vi "BASE-Main.vi"() -> ()   [LabVIEW 2017]
uses:
  <vilib>/Utility/error.llb/DialogType.ctl
  55ed0eea-cd20-493f-8468-85b8c1a0a0c0.vi
panel:
  out "Status Number":i32
  out "Status":i32(ring)=1 items=["Stopped"=1, "StartPending"=2, "StopPending"=3, "Running"=4, "ContinuePending"=5, "PausePending"=6, "Paused"=7]
  in  "RECIPE":bool
  out "error out":errorcluster
  in  "Logout":bool
  in  "Stop":bool
  in  "Create Login":bool
  in  "Reports":bool
  in  "Start":bool
  out "Time":string
  out "Date":string
  in  "Login":bool
  # "Machine Name"
  # "UNIQUE CIRCLE\nAUTOMATION Pvt Ltd"
types:
  T1 = enum8{"Enabled", "Disabled", "Disabled and Grayed Out"}
  T2 = typedef "DialogType.ctl" = u16
  T3 = enum32{"Invalid", "Standard", "Closed", "Hidden", "Minimized", "Maximized"}
  T4 = enum32{"invalid app kind", "Development System", "Run Time System", "Student Edition", "Embedded LabVIEW", "Evaluation", "Custom"}
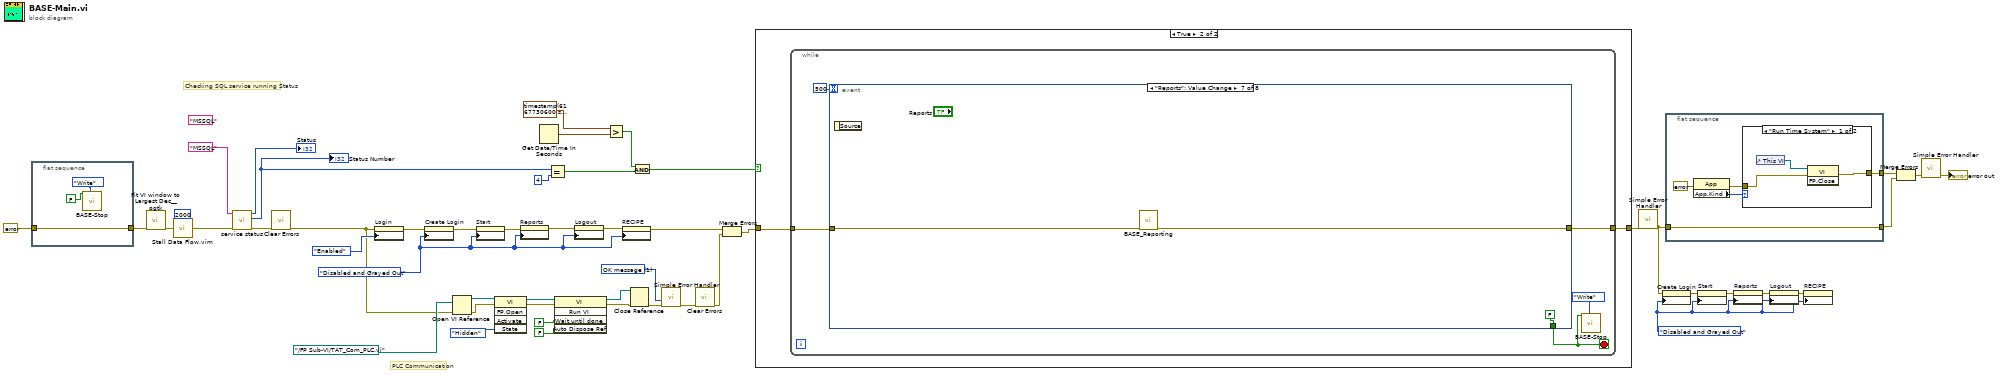
[diagram p0: block diagram]
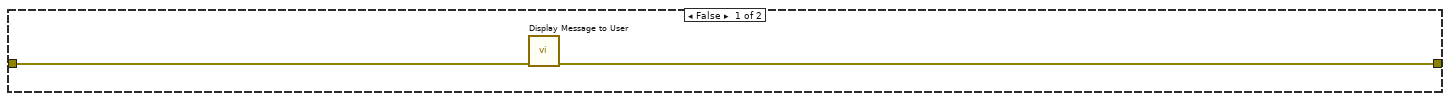
[diagram p3: hidden frame]
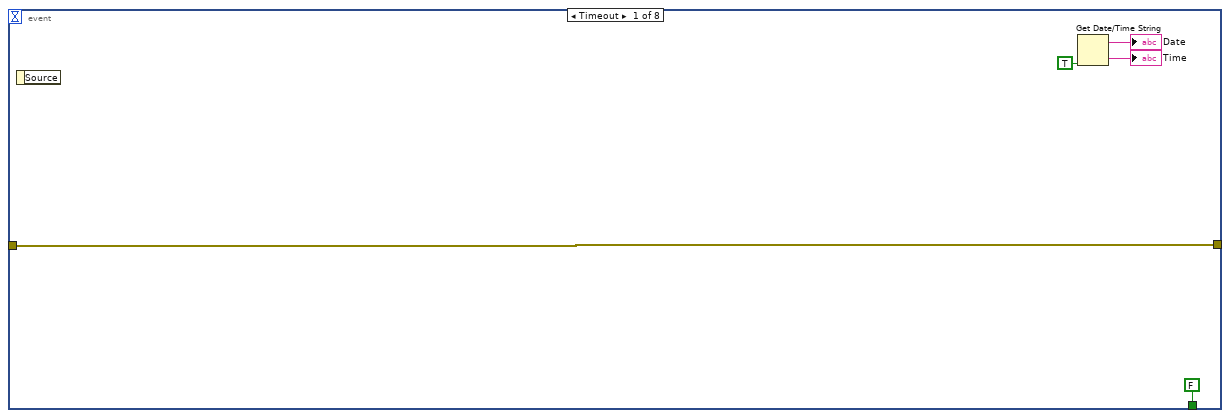
[diagram p4: hidden frame]
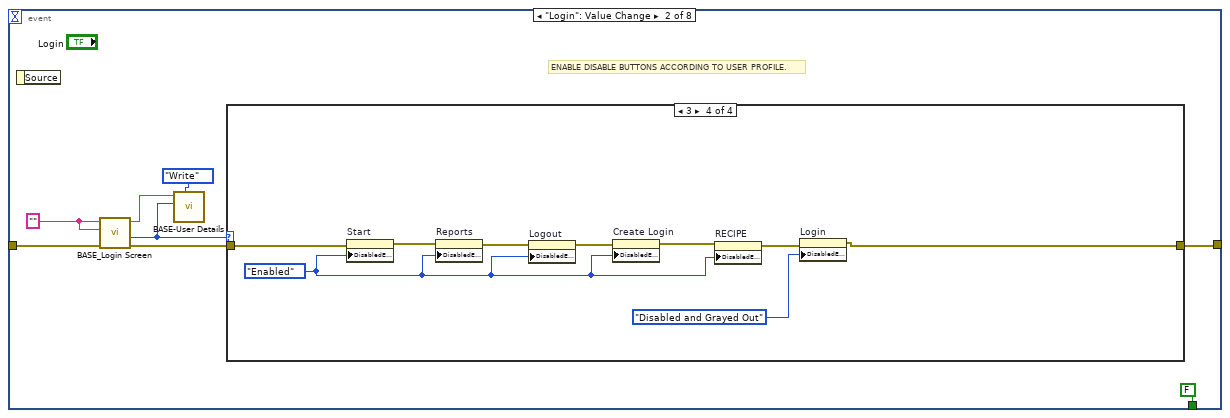
[diagram p5: hidden frame]
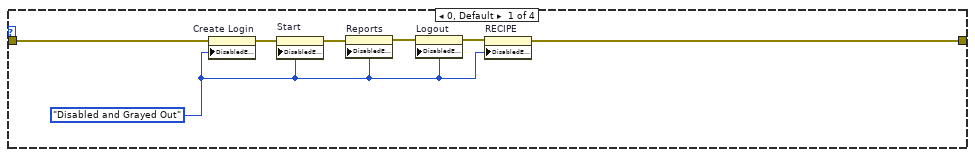
[diagram p6: hidden frame]
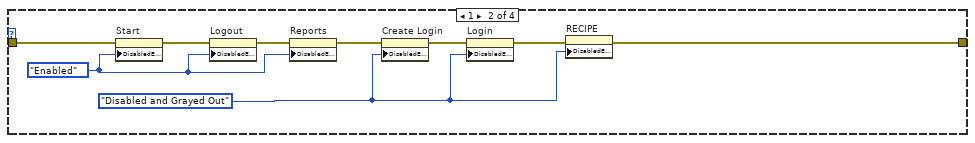
[diagram p7: hidden frame]
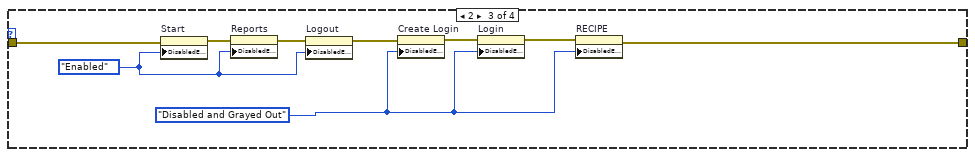
[diagram p8: hidden frame]
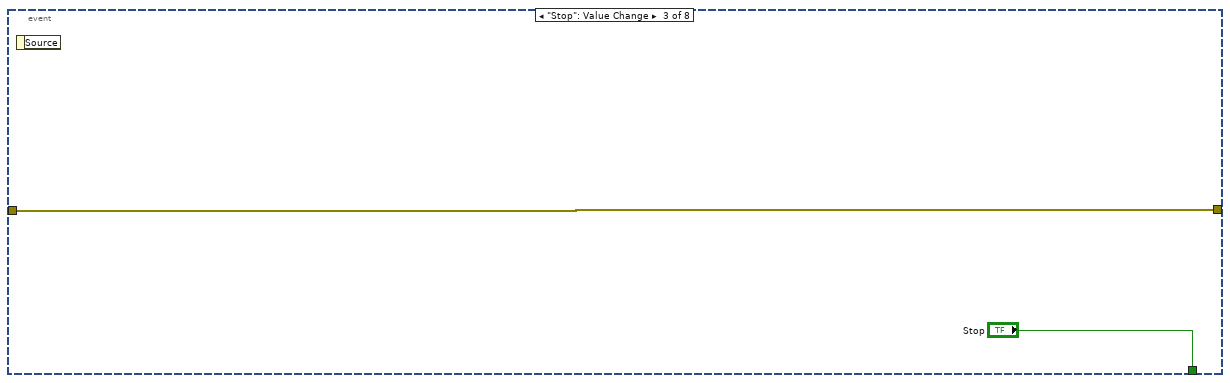
[diagram p9: hidden frame]
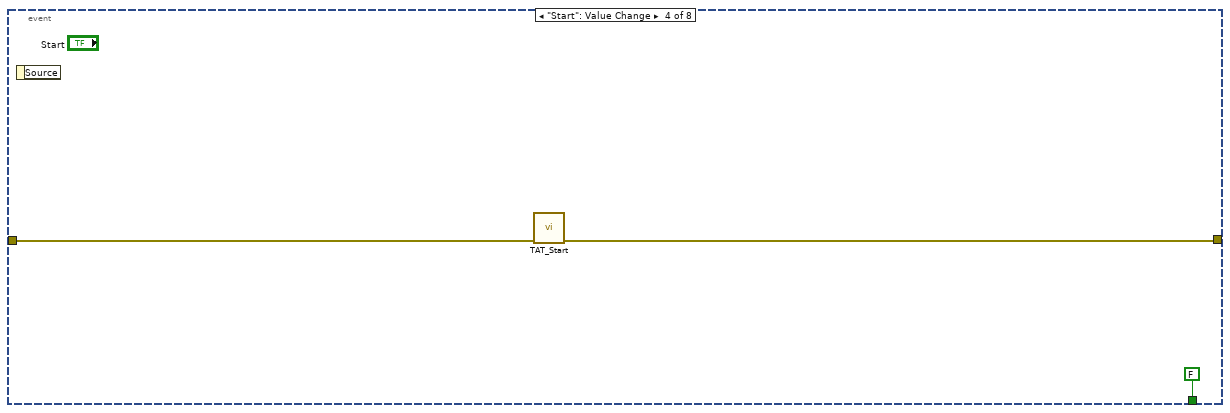
[diagram p10: hidden frame]
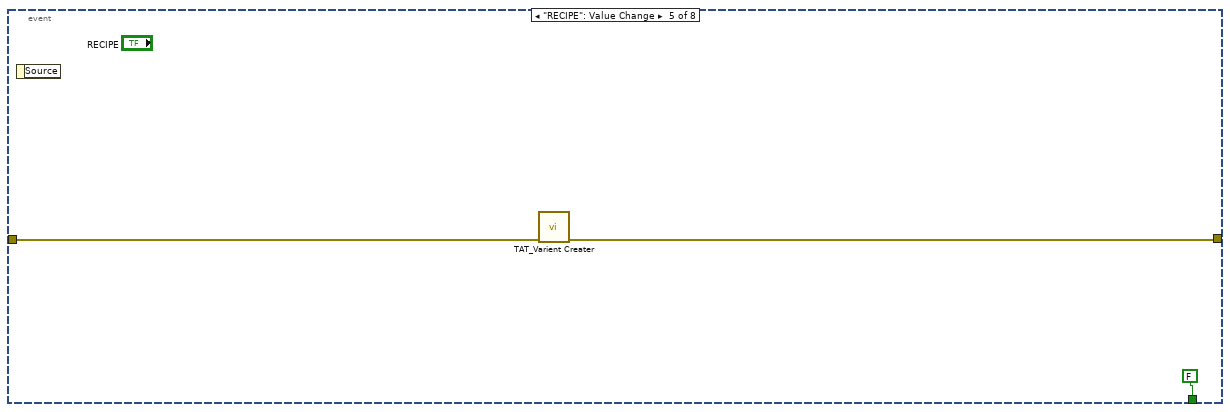
[diagram p11: hidden frame]
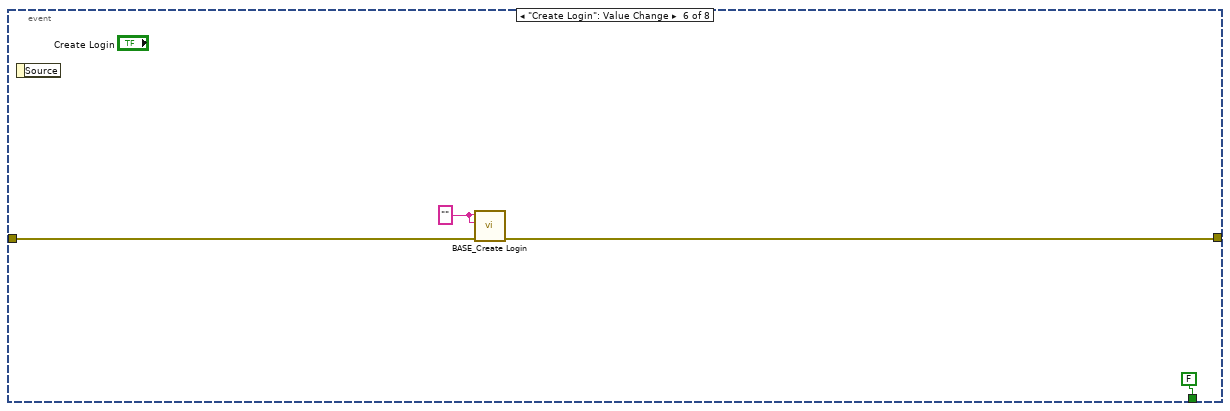
[diagram p12: hidden frame]
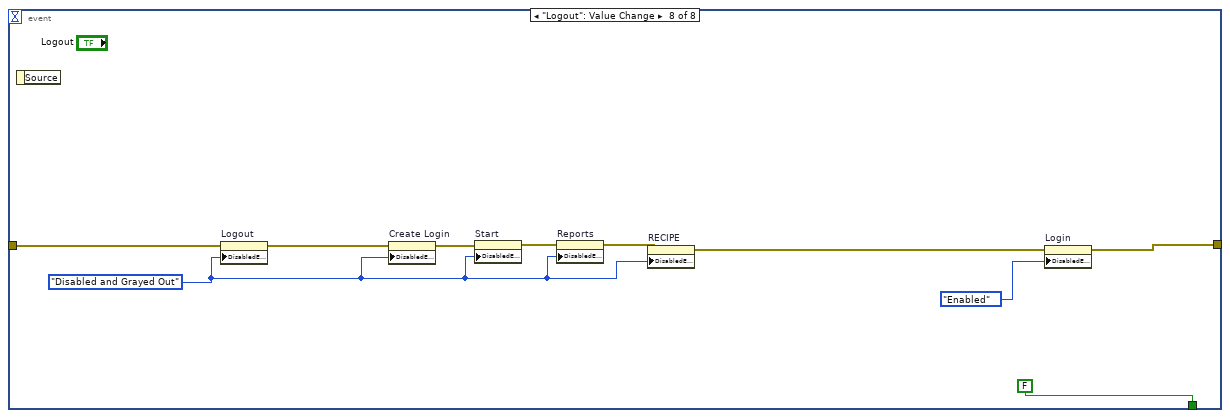
[diagram p13: hidden frame]
diagram:
  w7 = T1."Disabled and Grayed Out" ("Disabled")
  (unwired) "MSSQL" ("Service Name")
  w28 = T2 1 items=["no dialog", "OK message", "continue or stop message", "OK message + warnings", "continue/stop + warnings"] ("type of dialog (OK msg:1)")
  w8 = T1."Disabled and Grayed Out" ("Disabled")
  # "PLC Communication"
  # "Checking SQL service running Status"
  n1 = flat-sequence {
    tunnel: [w53] -> w41
    tunnel: errorcluster {"status"=FALSE, "code"=0, "source"=""} ("error constant") -> [w53]
    frame #0 {
      n2 = call "BASE-Stop.vi"("Enum"=enum16{"Read", "Write"}."Write", "Stop"=FALSE) -> ()  [unwired: 9 in, 1 out]
    }
  }
  n3 = call <userlib>:"Fit VI window to Largest Dec__ogtk.vi"("error in (no error)"=w41) -> ("error out"=w13:errorcluster)  [unwired: 5 in, 1 out]
  n4 = call "Stall Data Flow.vim"("value in"=w13, "milliseconds to wait"=u32 2000) -> ("value out"=w12:errorcluster)  [unwired: 1 out]
  n5 = call "service status.vi"("error in"=w12, "Service Name"="MSSQL") -> ("error out"=w20:errorcluster, "Status Number"=w22:i32, "Status"=→"Status":i32)  [unwired: 6 in, 1 out]
  "Status Number" <- w22
  n6 = call <vilib>:"Clear Errors.vi"("error in (no error)"=w20) -> ("error out"=w19:errorcluster)  [unwired: 5 in, 1 out]
  n7 = property on="Login" class="Bool"(error in=w19, "DisabledEnum"=T1."Enabled" ("Disabled")) -> (error out=w45:errorcluster)  [unwired: 1 in, 1 out]
  n8 = property on="Create Login" class="Bool"(error in=w45, "DisabledEnum"=w8) -> (error out=w49:errorcluster)  [unwired: 1 in, 1 out]
  n9 = Open VI Reference(vi path=path "../FP Sub-VI/TAT_Com_PLC.vi", error in (no error)=w19) -> (vi reference=w37:refnum<vi>, error out=w38:errorcluster)  [unwired: 4 in]
  n10 = property on="Start" class="Bool"(error in=w49, "DisabledEnum"=w8) -> (error out=w9:errorcluster)  [unwired: 1 in, 1 out]
  n11 = invoke class="VI" method="FP.Open"(reference=w37, error in=w38, "State"=T3."Hidden") -> (reference out=w40:refnum<vi>, error out=w39:errorcluster)  [unwired: 2 in, 3 out]
  n12 = property on="Reports" class="Bool"(error in=w9, "DisabledEnum"=w8) -> (error out=w43:errorcluster)  [unwired: 1 in, 1 out]
  n13 = Get Date/Time In Seconds() -> (seconds since 1Jan1904=w15:timestamp)
  n14 = Equal?(x=w22, y=4) -> (x = y?=w18:bool)
  n15 = invoke class="VI" method="Run VI"(reference=w40, error in=w39, "Wait until done"=FALSE ("Wait Until Done"), "Auto Dispose Ref"=FALSE ("Auto Dispose Reference")) -> (reference out=w36:refnum<vi>, error out=w35:errorcluster)  [unwired: 1 in, 3 out]
  n16 = property on="Logout" class="Bool"(error in=w43, "DisabledEnum"=w8) -> (error out=w10:errorcluster)  [unwired: 1 in, 1 out]
  n17 = Greater?(x=timestamp(6167730600 s since 1904-01-01), y=w15) -> (0:w14:bool)
  n18 = property on="RECIPE" class="Bool"(error in=w10, "DisabledEnum"=w8) -> (error out=w1:errorcluster)  [unwired: 1 in, 1 out]
  n19 = Close Reference(reference=w36, error in (no error)=w35) -> (error out=w29:errorcluster)
  n20 = And(x=w14, y=w18) -> (x .and. y?=w17:bool)
  n21 = call <vilib>:"Simple Error Handler.vi"("type of dialog (OK msg:1)"=w28, "error in (no error)"=w29) -> ("error out"=w27:errorcluster)  [unwired: 3 in, 4 out]
  n22 = call <vilib>:"Clear Errors.vi"("error in (no error)"=w27) -> ("error out"=w26:errorcluster)  [unwired: 5 in, 1 out]
  n23 = Merge Errors(w1, w26) -> (w31:errorcluster)
  n24 = case shown="True" w17 {
    tunnel: w31 -> [w55 w57]
    tunnel: [w54 w56] -> w50
    frame False {
      n25 = call "Display Message to User"("error in (no error)"=w55) -> ("error out"=w54:errorcluster)  [unwired: 9 in, 1 out]
    }
    frame True {
      n26 = while {
        tunnel: w57 -> [w61]
        tunnel: [w60] -> w56
        stop <- w58 stop-if-true
        n27 = event shown="[6] \"Reports\": Value Change" {
          selector: _ -> [_ _ _ _ _ _ _ _]
          dyn-events: _ -> [_ _ _ _ _ _ _ _]
          timeout: 500 -> [_ _ _ _ _ _ _ _]
          tunnel: w61 -> [w65 w75 w110 w113 w116 w121 w123 w131]
          tunnel: [w65 w68 w110 w112 w115 w120 w122 w132] -> w60
          tunnel: [FALSE ("Stop") FALSE ("Stop") "Stop" FALSE ("Stop") FALSE ("Stop") FALSE ("Stop") FALSE ("Stop") FALSE ("Stop")] -> w58
          event Timeout {
            n28 = event-data() -> ()  [unwired: 1 in, 1 out]
            n29 = Get Date/Time String(want seconds? (F)=TRUE) -> (date string=→"Date":string, time string=→"Time":string)  [unwired: 2 in]
          }
          event "Login": Value Change {
            w71 = "" ("User Name")
            # "ENABLE DISABLE BUTTONS ACCORDING TO USER PROFILE."
            n30 = event-data() -> ()  [unwired: 1 in, 1 out]
            n31 = call "BASE_Login Screen.vi"("Error In"=w75, "Password"=w71, "User Name"=w71) -> ("error out"=w74:errorcluster, "Level"=w69:i32, "User Name Out"=w72:string)  [unwired: 5 in, 1 out]
            n32 = call "BASE-User Details.vi"("Enum"=enum16{"Read", "Write"}."Write", "Level In"=w69, "User Name In"=w72) -> ()  [unwired: 7 in, 2 out]
            n33 = case shown="3" w69 {
              tunnel: w74 -> [w80 w91 w100 w109]
              tunnel: [w76 w83 w92 w101] -> w68
              frame 0, Default {
                w77 = T1."Disabled and Grayed Out" ("Disabled")
                n34 = property on="Create Login" class="Bool"(error in=w80, "DisabledEnum"=w77) -> (error out=w82:errorcluster)  [unwired: 1 in, 1 out]
                n35 = property on="Start" class="Bool"(error in=w82, "DisabledEnum"=w77) -> (error out=w81:errorcluster)  [unwired: 1 in, 1 out]
                n36 = property on="Reports" class="Bool"(error in=w81, "DisabledEnum"=w77) -> (error out=w78:errorcluster)  [unwired: 1 in, 1 out]
                n37 = property on="Logout" class="Bool"(error in=w78, "DisabledEnum"=w77) -> (error out=w79:errorcluster)  [unwired: 1 in, 1 out]
                n38 = property on="RECIPE" class="Bool"(error in=w79, "DisabledEnum"=w77) -> (error out=w76:errorcluster)  [unwired: 1 in, 1 out]
              }
              frame 1 {
                w85 = T1."Disabled and Grayed Out" ("Disabled")
                w84 = T1."Enabled" ("Disabled")
                n39 = property on="Start" class="Bool"(error in=w91, "DisabledEnum"=w84) -> (error out=w87:errorcluster)  [unwired: 1 in, 1 out]
                n40 = property on="Logout" class="Bool"(error in=w87, "DisabledEnum"=w84) -> (error out=w89:errorcluster)  [unwired: 1 in, 1 out]
                n41 = property on="Reports" class="Bool"(error in=w89, "DisabledEnum"=w84) -> (error out=w90:errorcluster)  [unwired: 1 in, 1 out]
                n42 = property on="Create Login" class="Bool"(error in=w90, "DisabledEnum"=w85) -> (error out=w88:errorcluster)  [unwired: 1 in, 1 out]
                n43 = property on="Login" class="Bool"(error in=w88, "DisabledEnum"=w85) -> (error out=w86:errorcluster)  [unwired: 1 in, 1 out]
                n44 = property on="RECIPE" class="Bool"(error in=w86, "DisabledEnum"=w85) -> (error out=w83:errorcluster)  [unwired: 1 in, 1 out]
              }
              frame 2 {
                w93 = T1."Disabled and Grayed Out" ("Disabled")
                w94 = T1."Enabled" ("Disabled")
                n45 = property on="Start" class="Bool"(error in=w100, "DisabledEnum"=w94) -> (error out=w97:errorcluster)  [unwired: 1 in, 1 out]
                n46 = property on="Reports" class="Bool"(error in=w97, "DisabledEnum"=w94) -> (error out=w99:errorcluster)  [unwired: 1 in, 1 out]
                n47 = property on="Logout" class="Bool"(error in=w99, "DisabledEnum"=w94) -> (error out=w95:errorcluster)  [unwired: 1 in, 1 out]
                n48 = property on="Create Login" class="Bool"(error in=w95, "DisabledEnum"=w93) -> (error out=w98:errorcluster)  [unwired: 1 in, 1 out]
                n49 = property on="Login" class="Bool"(error in=w98, "DisabledEnum"=w93) -> (error out=w96:errorcluster)  [unwired: 1 in, 1 out]
                n50 = property on="RECIPE" class="Bool"(error in=w96, "DisabledEnum"=w93) -> (error out=w92:errorcluster)  [unwired: 1 in, 1 out]
              }
              frame 3 {
                w102 = T1."Enabled" ("Disabled")
                n51 = property on="Start" class="Bool"(error in=w109, "DisabledEnum"=w102) -> (error out=w104:errorcluster)  [unwired: 1 in, 1 out]
                n52 = property on="Reports" class="Bool"(error in=w104, "DisabledEnum"=w102) -> (error out=w108:errorcluster)  [unwired: 1 in, 1 out]
                n53 = property on="Logout" class="Bool"(error in=w108, "DisabledEnum"=w102) -> (error out=w107:errorcluster)  [unwired: 1 in, 1 out]
                n54 = property on="Create Login" class="Bool"(error in=w107, "DisabledEnum"=w102) -> (error out=w106:errorcluster)  [unwired: 1 in, 1 out]
                n55 = property on="RECIPE" class="Bool"(error in=w106, "DisabledEnum"=w102) -> (error out=w105:errorcluster)  [unwired: 1 in, 1 out]
                n56 = property on="Login" class="Bool"(error in=w105, "DisabledEnum"=T1."Disabled and Grayed Out" ("Disabled")) -> (error out=w101:errorcluster)  [unwired: 1 in, 1 out]
              }
            }
          }
          event "Stop": Value Change {
            n57 = event-data() -> ()  [unwired: 1 in, 1 out]
          }
          event "Start": Value Change {
            n58 = event-data() -> ()  [unwired: 1 in, 1 out]
            n59 = call "TAT_Start.vi"("error In"=w113) -> ("error out"=w112:errorcluster)  [unwired: 10 in]
          }
          event "RECIPE": Value Change {
            n60 = event-data() -> ()  [unwired: 1 in, 1 out]
            n61 = call "TAT_Varient Creater.vi"("error in (no error)"=w116) -> ("error out"=w115:errorcluster)  [unwired: 10 in]
          }
          event "Create Login": Value Change {
            w119 = "" ("User Name")
            n62 = event-data() -> ()  [unwired: 1 in, 1 out]
            n63 = call "BASE_Create Login.vi"("Error In"=w121, "Password"=w119, "User Name"=w119) -> ("error out"=w120:errorcluster)  [unwired: 6 in]
          }
          event "Reports": Value Change {
            n64 = event-data() -> ()  [unwired: 1 in, 1 out]
            n65 = call "BASE_Reporting.vi"("error in (no error)"=w123) -> ("error out"=w122:errorcluster)  [unwired: 10 in]
          }
          event "Logout": Value Change {
            w126 = T1."Disabled and Grayed Out" ("Disabled")
            n66 = event-data() -> ()  [unwired: 1 in, 1 out]
            n67 = property on="Logout" class="Bool"(error in=w131, "DisabledEnum"=w126) -> (error out=w127:errorcluster)  [unwired: 1 in, 1 out]
            n68 = property on="Create Login" class="Bool"(error in=w127, "DisabledEnum"=w126) -> (error out=w134:errorcluster)  [unwired: 1 in, 1 out]
            n69 = property on="Start" class="Bool"(error in=w134, "DisabledEnum"=w126) -> (error out=w133:errorcluster)  [unwired: 1 in, 1 out]
            n70 = property on="Reports" class="Bool"(error in=w133, "DisabledEnum"=w126) -> (error out=w128:errorcluster)  [unwired: 1 in, 1 out]
            n71 = property on="RECIPE" class="Bool"(error in=w128, "DisabledEnum"=w126) -> (error out=w125:errorcluster)  [unwired: 1 in, 1 out]
            n72 = property on="Login" class="Bool"(error in=w125, "DisabledEnum"=T1."Enabled" ("Disabled")) -> (error out=w132:errorcluster)  [unwired: 1 in, 1 out]
          }
        }
        n73 = call "BASE-Stop.vi"("Enum"=enum16{"Read", "Write"}."Write", "Stop"=w58) -> ()  [unwired: 9 in, 1 out]
      }
    }
  }
  n74 = call <vilib>:"Simple Error Handler.vi"("error in (no error)"=w50) -> ("error out"=w2:errorcluster)  [unwired: 4 in, 4 out]
  n75 = property on="Create Login" class="Bool"(error in=w2, "DisabledEnum"=w7) -> (error out=w3:errorcluster)  [unwired: 1 in, 1 out]
  n76 = flat-sequence {
    tunnel: [w136] -> w48
    tunnel: [w135] -> w46
    tunnel: w2 -> [w135]
    frame #0 {
      n77 = property class="App"(error in=errorcluster {"status"=FALSE, "code"=0, "source"=""} ("error in (no error)")) -> (error out=w138:errorcluster, "App.Kind"=w139:T4)  [unwired: 1 in, 1 out]
      n78 = case shown="\"Run Time System\"" w139 {
        tunnel: w138 -> [w141 w143]
        tunnel: [w140 w143] -> w136
        frame "Run Time System" {
          n79 = control-ref of="This VI"() -> (w142:refnum<vi>)
          n80 = invoke class="VI" method="FP.Close"(reference=w142, error in=w141) -> (error out=w140:errorcluster)  [unwired: 1 in, 2 out]
        }
        frame "Development System", Default {
        }
      }
    }
  }
  n81 = property on="Start" class="Bool"(error in=w3, "DisabledEnum"=w7) -> (error out=w6:errorcluster)  [unwired: 1 in, 1 out]
  n82 = property on="Reports" class="Bool"(error in=w6, "DisabledEnum"=w7) -> (error out=w4:errorcluster)  [unwired: 1 in, 1 out]
  n83 = property on="Logout" class="Bool"(error in=w4, "DisabledEnum"=w7) -> (error out=w5:errorcluster)  [unwired: 1 in, 1 out]
  n84 = property on="RECIPE" class="Bool"(error in=w5, "DisabledEnum"=w7) -> ()  [unwired: 1 in, 2 out]
  n85 = Merge Errors(w48, w46) -> (w47:errorcluster)
  n86 = call <vilib>:"Simple Error Handler.vi"("error in (no error)"=w47) -> ("error out"=→"error out":errorcluster)  [unwired: 4 in, 4 out]
